vi "Custom Error Manager.vi"(5 "Code":i32, 6 "Mode":T1(ring)=enum."Add Errors", 7 "Description":string, 8 "error in (no error)":errorcluster, 11 "Custom Error Code Path":path=path "C:/programdata/crystaldetect/errorcodes.ini") -> (0 "error out":errorcluster, 3 "Error String":string)   [LabVIEW 2017]
uses:
  <vilib>/Utility/error.llb/DialogType.ctl
  <vilib>/Utility/config.llb/Write Key (String).vi
  <vilib>/Utility/config.llb/NI_LVConfig.lvlib
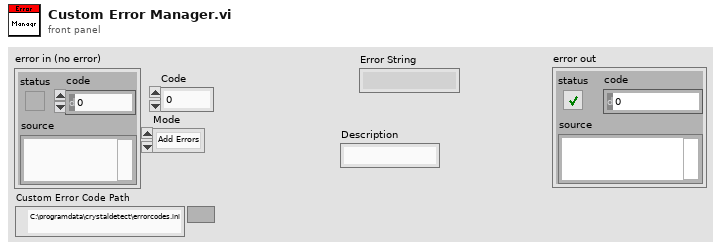
[diagram p1: front panel]
types:
  T1 = enum16{"NULL", "Load Errors", "Add Errors", "Process Error"}
  T2 = typedef "NI_LVConfig.lvlib/Config Data RefNum.ctl" = refnum<k1>
  T3 = typedef "DialogType.ctl" = u16
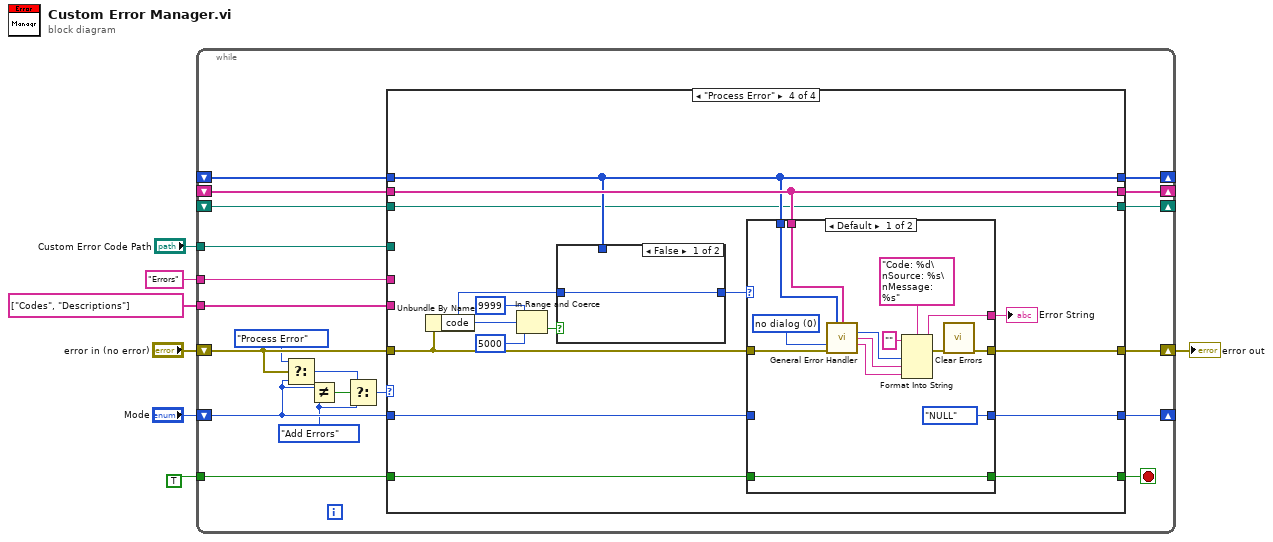
[diagram p0: block diagram]
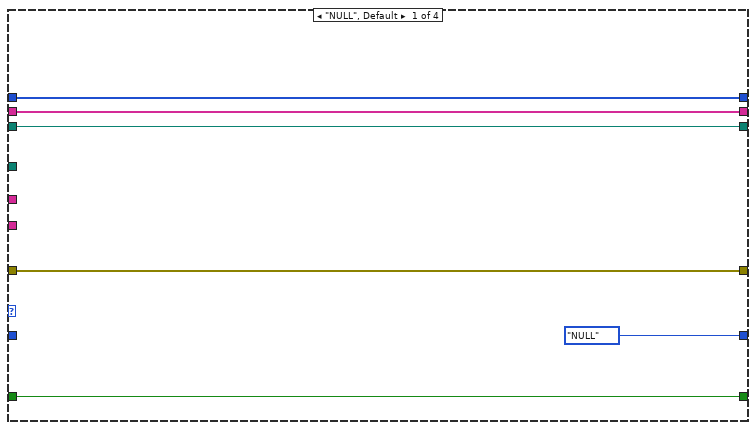
[diagram p2: hidden frame]
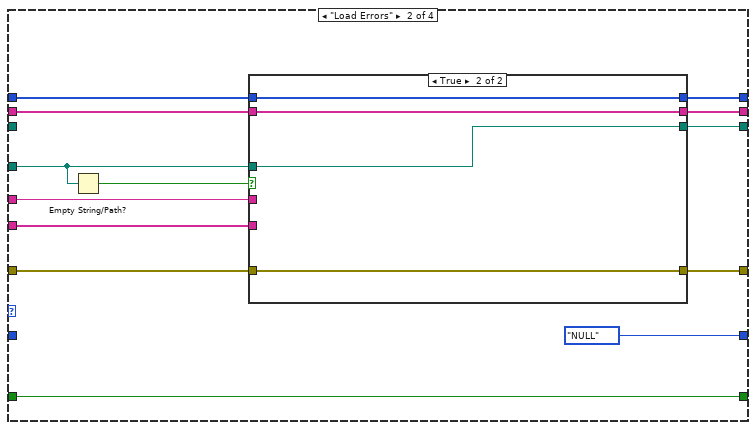
[diagram p3: hidden frame]
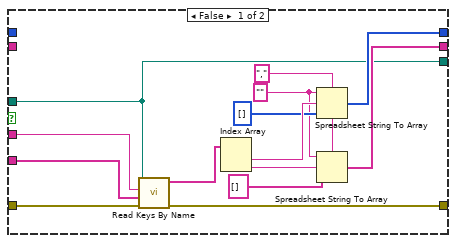
[diagram p4: hidden frame]
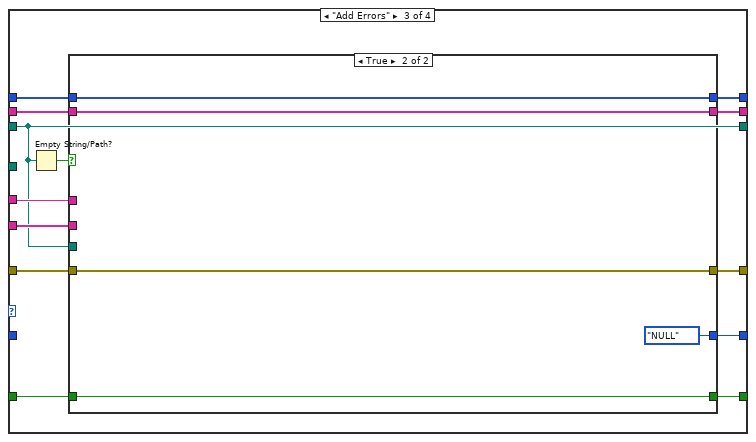
[diagram p5: hidden frame]
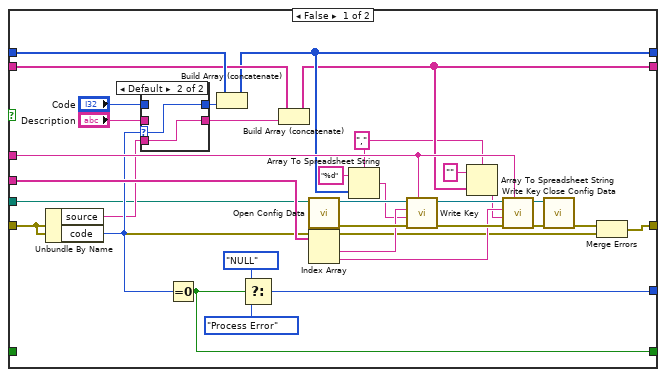
[diagram p6: hidden frame]
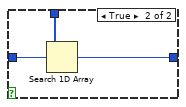
[diagram p8: hidden frame]
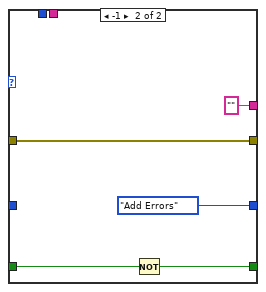
[diagram p9: hidden frame]
diagram:
  n1 = while {
    shift-right: [w24] -> _
    shift-left: _ -> [w23]
    shift-right: [w25] -> _
    shift-left: _ -> [w22]
    tunnel: "Errors" ("section") -> [w26]
    tunnel: string[] ["Codes", "Descriptions"] ("array type (2D Dbl)") -> [w21]
    shift-right: [w27] -> w6
    shift-left: "error in (no error)" -> [w20]
    shift-right: [w18] -> _
    shift-left: "Mode" -> [w17]
    shift-right: [w12] -> _
    shift-left: _ -> [w11]
    tunnel: TRUE -> [w10]
    tunnel: "Custom Error Code Path" -> [w8]
    stop <- w9 stop-if-true
    w15 = T1."Add Errors"
    n2 = Select(t=T1."Process Error", s=w20, f=w17) -> (s? t:f=w14:T1)
    n3 = Not Equal?(x=w17, y=w15) -> (x != y?=w16:bool)
    n4 = Select(t=w14, s=w16, f=w15) -> (s? t:f=w13:T1)
    n5 = case shown="\"Process Error\"" w13 {
      tunnel: w20 -> [w33 w46 w69 w132]
      tunnel: [w33 w45 w70 w134] -> w27
      tunnel: w26 -> [_ w44 w77 _]
      tunnel: [w31 w43 w72 w133] -> w25
      tunnel: [w32 w42 w73 w131] -> w24
      tunnel: w23 -> [w32 w36 w76 w131]
      tunnel: w22 -> [w31 w35 w75 w133]
      tunnel: w21 -> [_ w41 w74 _]
      tunnel: w17 -> [_ _ _ w129]
      tunnel: [T1."NULL" T1."NULL" w71 w128] -> w18
      tunnel: [w29 w34 w66 w127] -> w12
      tunnel: w11 -> [w29 _ w66 w127]
      tunnel: w10 -> [w28 w39 w65 w126]
      tunnel: [w28 w39 w68 w125] -> w9
      tunnel: w8 -> [_ w38 _ _]
      frame "NULL", Default {
      }
      frame "Load Errors" {
        n6 = Empty String/Path?(string/path=w38) -> (empty?=w37:bool)
        n7 = case shown="True" w37 {
          tunnel: w46 -> [w60 w62]
          tunnel: [w59 w62] -> w45
          tunnel: w44 -> [w58 _]
          tunnel: [w51 w63] -> w43
          tunnel: [w50 w64] -> w42
          tunnel: w41 -> [w49 _]
          tunnel: w38 -> [w47 w61]
          tunnel: w36 -> [_ w64]
          tunnel: w35 -> [_ w63]
          tunnel: [w47 w61] -> w34
          frame False {
            w48 = "" ("format string")
            w53 = "," ("delimiter (Tab)")
            n8 = call "Read Keys By Name.vi"("error in (no error)"=w60, "Search Keys"=w49, "section"=w58, "Hardware INI Path"=w47) -> ("error out"=w59:errorcluster, "Key Data"=w57:string[])  [unwired: 6 in]
            n9 = Index Array(array=w57) -> (element #1=w56:string, element #2=w54:string)  [unwired: 2 in]
            n10 = Spreadsheet String To Array(delimiter (Tab)=w53, format string=w48, spreadsheet string=w56, array type (2D Dbl)=i32[] [] ("[user-defined codes]")) -> (array=w50:i32[])
            n11 = Spreadsheet String To Array(delimiter (Tab)=w53, format string=w48, spreadsheet string=w54, array type (2D Dbl)=string[] []) -> (array=w51:string[])
          }
          frame True {
          }
        }
      }
      frame "Add Errors" {
        n12 = Empty String/Path?(string/path=w66) -> (empty?=w67:bool)
        n13 = case shown="True" w67 {
          tunnel: w77 -> [w104 _]
          tunnel: w76 -> [w103 w119]
          tunnel: w75 -> [w102 w118]
          tunnel: w74 -> [w101 _]
          tunnel: [w98 w119] -> w73
          tunnel: [w96 w118] -> w72
          tunnel: [w89 T1."NULL"] -> w71
          tunnel: w66 -> [w82 _]
          tunnel: [w81 w117] -> w70
          tunnel: w69 -> [w80 w117]
          tunnel: [w79 w115] -> w68
          tunnel: w65 -> [_ w115]
          frame False {
            w94 = "," ("delimiter (Tab)")
            n14 = Unbundle By Name(w80) -> ("source"=w83:string, "code"=w88:i32)
            n15 = case shown="Default" w88 {
              selector: w88 -> [_ w114]
              tunnel: "Code" -> [w112 _]
              tunnel: [w112 w114] -> w86
              tunnel: [w111 w113] -> w85
              tunnel: "Description" -> [w111 _]
              tunnel: w83 -> [_ w113]
              frame 0 {
              }
              frame Default {
              }
            }
            n16 = Equal To 0?(x=w88) -> (x = 0?=w79:bool)
            n17 = Build Array (concatenate)(w103, w86) -> (w98:i32[])
            n18 = Select(t=T1."NULL", s=w79, f=T1."Process Error") -> (s? t:f=w89:T1)
            n19 = Build Array (concatenate)(w102, w85) -> (w96:string[])
            n20 = call <vilib>:"Open Config Data.vi"("configuration file path"=w82) -> ("error out"=w105:errorcluster, "refnum"=w106:T2)  [unwired: 8 in, 1 out]
            n21 = Index Array(array=w101) -> (element #1=w100:string, element #2=w99:string)  [unwired: 2 in]
            n22 = Array To Spreadsheet String(delimiter (Tab)=w94, array=w98, 3:"%d" ("format string")) -> (spreadsheet string=w97:string)
            n23 = call-poly <vilib>:"Write Key.vi"("section"=w104, "error in (no error)"=w105, "value"=w97, "key"=w100, "refnum"=w106) -> ("error out"=w110:errorcluster, "refnum out"=w109:T2)  [unwired: 4 in, 1 out]
            n24 = Array To Spreadsheet String(delimiter (Tab)=w94, array=w96, 3:"" ("format string")) -> (spreadsheet string=w93:string)
            n25 = call-poly <vilib>:"Write Key.vi"("section"=w104, "error in (no error)"=w110, "value"=w93, "key"=w99, "refnum"=w109) -> ("error out"=w108:errorcluster, "refnum out"=w107:T2)  [unwired: 4 in, 1 out]
            n26 = call <vilib>:"Close Config Data.vi"("error in (no error)"=w108, "refnum"=w107) -> ("error out"=w92:errorcluster)  [unwired: 8 in, 1 out]
            n27 = Merge Errors(w92, w80) -> (w81:errorcluster)
          }
          frame True {
          }
        }
      }
      frame "Process Error" {
        n28 = Unbundle By Name(w132) -> ("code"=w121:i32)
        n29 = In Range and Coerce(upper limit=9999, x=w121, lower limit=5000) -> (In Range?=w120:bool)  [unwired: 1 out]
        n30 = case shown="False" w120 {
          tunnel: w131 -> [_ w138]
          tunnel: [w135 w137] -> w130
          tunnel: w121 -> [w135 w136]
          frame False {
          }
          frame True {
            n31 = Search 1D Array(1D array=w138, element=w136) -> (index of element=w137:i32)  [unwired: 1 in]
          }
        }
        n32 = case shown="Default" w130 {
          tunnel: [w139 w157] -> w134
          tunnel: w133 -> [w151 _]
          tunnel: w132 -> [w150 w157]
          tunnel: w131 -> [w149 _]
          tunnel: w129 -> [_ _]
          tunnel: [T1."NULL" T1."Add Errors"] -> w128
          tunnel: w126 -> [w147 w155]
          tunnel: [w147 w154] -> w125
          tunnel: [w140 ""] -> w124
          frame Default {
            w152 = T3 0 items=["no dialog", "OK message", "continue or stop message", "OK message + warnings", "continue/stop + warnings"] ("type of dialog (OK msg:1)")
            n33 = call <vilib>:"General Error Handler.vi"("[user-defined codes]"=w149, "[user-defined descriptions]"=w151, "type of dialog (OK msg:1)"=w152, "error in (no error)"=w150) -> ("code out"=w145:i32, "source out"=w144:string, "message"=w143:string)  [unwired: 7 in, 2 out]
            n34 = Format Into String(format string="Code: %d\nSource: %s\nMessage: %s", initial string="", w145, w144, w143) -> (resulting string=w140:string, error out=w146:errorcluster)  [unwired: 1 in]
            n35 = call <vilib>:"Clear Errors.vi"("error in (no error)"=w146) -> ("error out"=w139:errorcluster)  [unwired: 5 in, 1 out]
          }
          frame -1 {
            n36 = Not(x=w155) -> (.not. x?=w154:bool)
          }
        }
        "Error String" <- w124
      }
    }
  }
  "error out" <- w6
